vi "RecordAvgVolts.vi"() -> (5 "Plug in titles":string[](array[string]), 7 "Plug in values":string[](array[string]))   [LabVIEW 2021]
uses:
  <vilib>/Analysis/baseanly.llb/Mean (DBL).vi
  Globals/Meas_global.vi
  <vilib>/Analysis/NI_AALBase.lvlib
panel:
  out "perBlockMeanV":dbl[][](array[numeric])
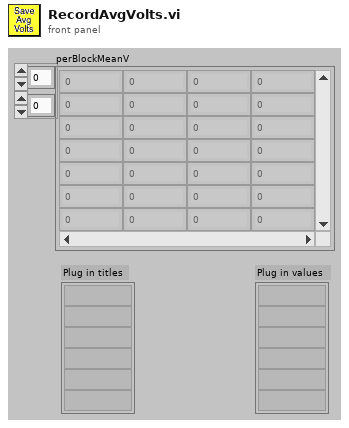
[diagram p1: front panel]
types:
  T1 = typedef "Time_Trace_Cluster.ctl" = cluster{"Weighting":dbl[], "Voltage":dbl[], "Eng Values":dbl[]}
  T2 = typedef "Analysis_info_cluster.ctl" = cluster{"Colour":u32, "Inst type":T3, "Inst name":string, "Symbol":string, "Code name":string, "Extra Info":string, "Inst Array":T4, "Extra Titles":string[], "Extra Values":string[], "U":dbl, "u^2":dbl, "u^3":dbl, "u^4":dbl, "Skew_u":dbl, "Kurt_u":dbl, "Sd Error in Mean":dbl, "% u'/U":dbl, "X":dbl, "Y":dbl, "Z":dbl, "Timescale integral Estimate":dbl, "Sd Error in Variance":dbl, "Calib File":path, "Calib Constants":dbl[], "Output Position":bool, "Stats":enum16{"None", "Basic", "Full"}, "Av Sampling Rate":dbl, "Av No of Samples":dbl, "Total Meas Time (s)":dbl, "ADAM Ch Name":string, "Max value":dbl, "Min value":dbl, "Req Sample Rate Hz":dbl, "Sync Delay Time (s)":dbl, "Ch No":i16, "Device":string, "Use Latest Calib":bool, "Port":string, "Metadata Ch Names":string[], "Metadata Ch Values":string[], "Label":string}
  T3 = typedef "Inst_type.ctl" = enum16{"Raw voltage", "Raw with zero offsetting", "Propeller anemometer", "Pressure Transducer", "Pitot-static tube", "Hot wire", "Cross wire 1", "Cross wire 2", "Generic Linear", "Generic Polynomial", "Generic BackPoly", "Fast FID", "Thermocouple", "Cold wire", "Pulsed Wire", "LDA Vel", "LDA Tran time", "LDA Arr time", "Microphone"}
  T4 = typedef "Instrument_Array.ctl" = enum16{"PWA", "LDA", "Analogue"}
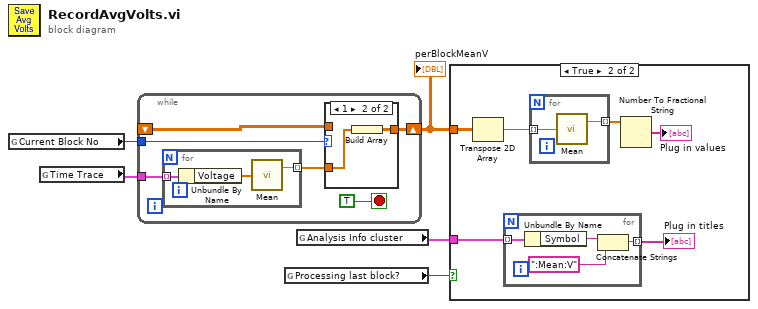
[diagram p0: block diagram]
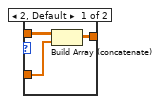
[diagram p3: hidden frame]
diagram:
  n1 = global read "Meas_global.vi" "Current Block No"() -> (w4:i32)
  n2 = global read "Meas_global.vi" "Time Trace"() -> (w5:T1[])
  n3 = while {
    tunnel: w5 -> [w11]
    shift-right: [w8] -> w1
    shift-left: _ -> [w6]
    tunnel: w4 -> [w9]
    stop <- TRUE stop-if-true
    n4 = for {
      tunnel: w11 -> [w18] mode=indexing
      tunnel: [w17] -> w7 mode=indexing
      n5 = Unbundle By Name(w18) -> ("Voltage"=w19:dbl[])
      n6 = call-poly <vilib>:"Mean.vi"("X"=w19) -> ("mean"=w17:dbl)  [unwired: 1 out]
    }
    n7 = case shown="1" w9 {
      tunnel: [w14 w15] -> w8
      tunnel: w7 -> [w13 w16]
      tunnel: w6 -> [w12 _]
      frame 2, Default {
        n8 = Build Array (concatenate)(w12, w13) -> (w14:dbl[][])
      }
      frame 1 {
        n9 = Build Array(w16) -> (w15:dbl[][])
      }
    }
  }
  "perBlockMeanV" <- w1
  n10 = global read "Meas_global.vi" "Processing last block?"() -> (w3:bool)
  n11 = global read "Meas_global.vi" "Analysis Info cluster"() -> (w2:T2[])
  n12 = case shown="True" w3 {
    tunnel: w2 -> [_ w24]
    tunnel: w1 -> [_ w23]
    frame False {
    }
    frame True {
      n13 = Transpose 2D Array(2D array=w23) -> (transposed array=w20:dbl[][])
      n14 = for {
        tunnel: w24 -> [w31] mode=indexing
        tunnel: [w28] -> w25 mode=indexing
        n15 = Unbundle By Name(w31) -> ("Symbol"=w30:string)
        n16 = Concatenate Strings(w30, ":Mean:V" ("string")) -> (w28:string)
      }
      "Plug in titles" <- w25
      n17 = for {
        tunnel: w20 -> [w27] mode=indexing
        tunnel: [w26] -> w22 mode=indexing
        n18 = call-poly <vilib>:"Mean.vi"("X"=w27) -> ("mean"=w26:dbl)  [unwired: 1 out]
      }
      n19 = Number To Fractional String(number=w22) -> (F-format string=→"Plug in values":string[])  [unwired: 3 in]
    }
  }
